vi "mlink_ai_scan .vi"(6 "Channels":u8[](array[numeric]), 8 "error in (no error)":errorcluster, 9 "timeout":i32, 10 "scan count":i32, 11 "connection ID":i32=-1) -> (0 "error out":errorcluster, 1 "read samples":i32, 2 "Values":dbl[][](array[numeric]), 3 "connection ID out":i32)   [LabVIEW 2009, in "MicroDAQ.lvlib" / "mlink.lvlib"]
doc: "This function starts analog input scanning session and reads acquired data. The function call has to be preceded with mlink_ai_scan_init() which initiates scanning session parameters. The scan_count argument determines how many scans function will read. If scan_count argument is 0 function will start data acquisistion without waiting for data. The timeout argument \nspecifies the amount of time in miliseconds to wait for samples to become available. If the\ntime elapses, the runction returns a negative value and any samples read before the timeout elapsed. If timeout is set to -1, the function waits indefinitely. If timeout is set to 0, the\nfunction tries once to read the requested samples and returns number of scans read by function call. The number of acquired scans is returned by function. Values of acquired data is returned as an m-by-n array, where m is the number of acquired scans, and n is the number of used\ninput channels (defined during initialization with mlink_ai_scan_init() function call)."
uses:
  <instrlib>/MicroDAQ/Mlink library wraper/mlink.lvlib
  <instrlib>/MicroDAQ/MLink32.dll
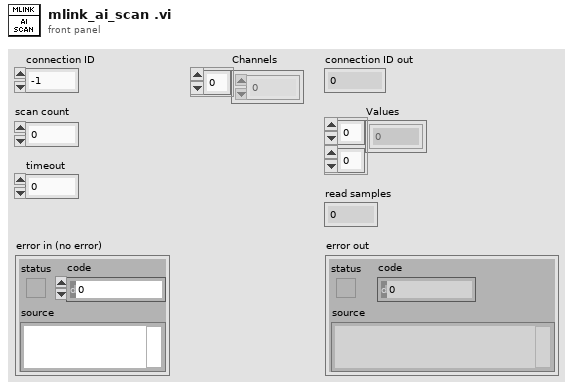
[diagram p1: front panel]
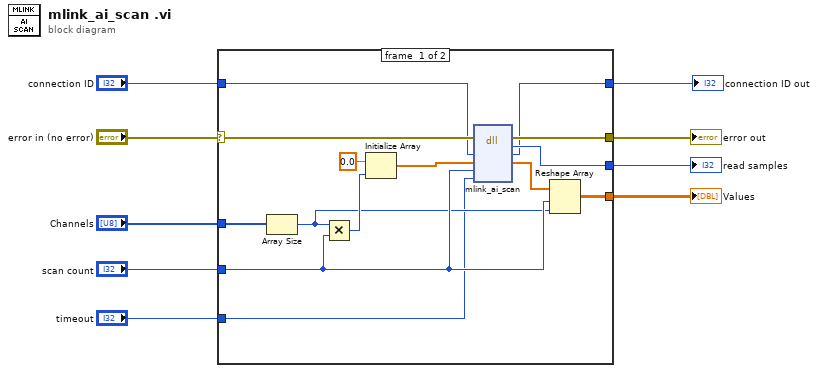
[diagram p0: block diagram]
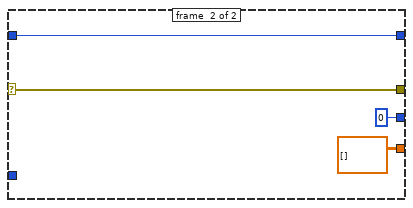
[diagram p2: hidden frame]
diagram:
  n1 = case shown="No Error" "error in (no error)" {
    selector: "error in (no error)" -> [w23 w26]
    tunnel: "scan count" -> [w18 _]
    tunnel: [w16 0 ("return type")] -> w7
    tunnel: "Channels" -> [w15 _]
    tunnel: [w14 dbl[][] [] ("data")] -> w5
    tunnel: [w13 w26] -> w4
    tunnel: "connection ID" -> [w12 w27]
    tunnel: [w11 w27] -> w2
    tunnel: "timeout" -> [w10 _]
    frame #0 {
      n2 = Array Size(array=w15) -> (size(s)=w17:i32)
      n3 = Multiply(x=w17, y=w18) -> (x*y=w20:i32)
      n4 = Initialize Array(0.0 ("element"), w20) -> (w22:dbl[])
      n5 = dll-call lib="C:/Program Files (x86)/National Instruments/LabVIEW 2009/instr.lib/MicroDAQ/MLink32.dll" fn="mlink_ai_scan"(error in=w23, "link_fd"=w12, "data"=w22, "scan count"=w18, "timeout"=w10) -> (error out=w13:errorcluster, "return type"=w16:i32, "link_fd"=w11:i32, "data"=w19:dbl[])  [unwired: 4 in, 1 out]
      n6 = Reshape Array(w19, w18, w17) -> (w14:dbl[][])
    }
    frame #1 {
    }
  }
  "connection ID out" <- w2
  "error out" <- w4
  "read samples" <- w7
  "Values" <- w5
